vi "specu1a 1.0.0 Write User EEPROM.vi"(0 "Device Handle":i32, 1 "Address":u16, 2 "EEPROM String in":string, 3 "error in (no error)":errorcluster, 4 "Length":u16=256) -> (5 "Device Handle out":i32, 6 "EEPROM String out":string, 7 "error out":errorcluster)   [LabVIEW 2010]
uses:
  WINDOWS/SYSTEM32/DRIVERS/specu1a.dll
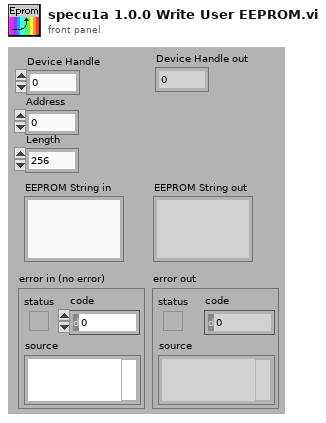
[diagram p1: front panel]
types:
  T1 = cluster{"[0]":u8, "[1]":u8, "[2]":u8, "[3]":u8, "[4]":u8, "[5]":u8, "[6]":u8, "[7]":u8, "[8]":u8, "[9]":u8, "[10]":u8, "[11]":u8, "[12]":u8, "[13]":u8, "[14]":u8, "[15]":u8, "[16]":u8, "[17]":u8, "[18]":u8, "[19]":u8, "[20]":u8, "[21]":u8, "[22]":u8, "[23]":u8, "[24]":u8, "[25]":u8, "[26]":u8, "[27]":u8, "[28]":u8, "[29]":u8, "[30]":u8, "[31]":u8, "[32]":u8, "[33]":u8, "[34]":u8, "[35]":u8, "[36]":u8, "[37]":u8, "[38]":u8, "[39]":u8, "[40]":u8, "[41]":u8, "[42]":u8, "[43]":u8, "[44]":u8, "[45]":u8, "[46]":u8, "[47]":u8, "[48]":u8, "[49]":u8, "[50]":u8, "[51]":u8, "[52]":u8, "[53]":u8, "[54]":u8, "[55]":u8, "[56]":u8, "[57]":u8, "[58]":u8, "[59]":u8, "[60]":u8, "[61]":u8, "[62]":u8, "[63]":u8}
  T2 = typedef "specu1a 1.0.0 Error codes.ctl" = enum16{"INVALID_HANDLE_VALUE", "USBDEV_SUCCESS", "USBDEV_INVALID_HANDLE", "USBDEV_UNSUCCESS", "USBDEV_INVALID_VALUE", "USBDEV_CHECK_NORMAL", "USBDEV_CHECK_INVALID", "USBDEV_CHECK_REMOVE", "USBDEV_CHECK_OTHER", "USBDEV_RESET_ERROR", "USBDEV_BULKSIZE_ERROR", "USBDEV_BULK_READ_ERROR", "USBDEV_BULK_NOT_UPDATED", "USBDEV_TIME_OVER_ERROR", "USBDEV_TIME_UNDER_ERROR", "USBDEV_TIME_SET_ERROR", "USBDEV_SET_GAIN_ERROR", "USBDEV_GET_TEMP_ERROR", "USBDEV_SET_TRIGGER_ERROR", "USBDEV_RW_EEP_ADDR_ERROR", "USBDEV_RW_EEP_SIZE_ERROR", "USBDEV_RW_EEP_OVER_ERROR", "USBDEV_RW_EEP_ERROR", "UNITID_PRODUCTID_CONFLICT", "UNKNOWN_ERROR"}
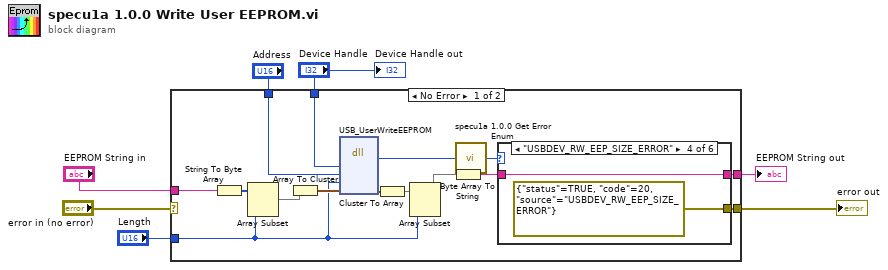
[diagram p0: block diagram]
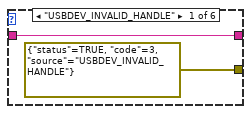
[diagram p2: hidden frame]
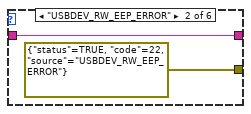
[diagram p3: hidden frame]
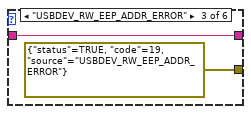
[diagram p4: hidden frame]
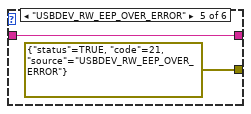
[diagram p5: hidden frame]
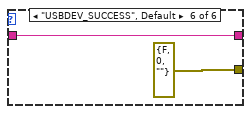
[diagram p6: hidden frame]
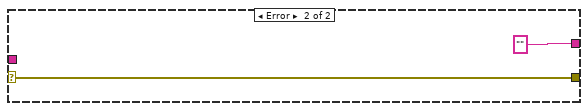
[diagram p7: hidden frame]
diagram:
  n1 = case shown="No Error" "error in (no error)" {
    selector: "error in (no error)" -> [_ w36]
    tunnel: [w21 w36] -> w6
    tunnel: "Device Handle" -> [w16 _]
    tunnel: "Address" -> [w15 _]
    tunnel: "Length" -> [w8 _]
    tunnel: [w17 "" ("string")] -> w1
    tunnel: "EEPROM String in" -> [w10 _]
    frame No Error {
      n2 = String To Byte Array(string=w10) -> (unsigned byte array=w11:u8[])
      n3 = Array Subset(array=w11, length=w8) -> (w9:u8[])  [unwired: 1 in]
      n4 = Array To Cluster(array=w9) -> (cluster=w14:T1)
      n5 = dll-call lib="C:/WINDOWS/SYSTEM32/DRIVERS/specu1a.dll" fn="USB_UserWriteEEPROM" label="1.0.0 Write User EEPROM"("Device Handle"=w16, "Address"=w15, "Length"=w8, w14) -> (w13:u16, w12:T1)  [unwired: 6 in, 2 out]
      n6 = Cluster To Array(cluster=w12) -> (array=w20:u8[])
      n7 = Array Subset(array=w20, length=w8) -> (w19:u8[])  [unwired: 1 in]
      n8 = Byte Array To String(unsigned byte array=w19) -> (string=w18:string)
      n9 = call "specu1a 1.0.0 Get Error Enum.vi"("Error Code in"=w13) -> ("Specu1a 1.0.0 Error code out"=w22:T2)  [unwired: 4 in]
      n10 = case shown="\"USBDEV_RW_EEP_SIZE_ERROR\"" w22 {
        tunnel: [w23 w25 w27 w29 w31 w33] -> w17
        tunnel: [errorcluster {"status"=TRUE, "code"=3, "source"="USBDEV_INVALID_HANDLE"} ("error out") errorcluster {"status"=TRUE, "code"=22, "source"="USBDEV_RW_EEP_ERROR"} ("error out") errorcluster {"status"=TRUE, "code"=19, "source"="USBDEV_RW_EEP_ADDR_ERROR"} ("error out") errorcluster {"status"=TRUE, "code"=20, "source"="USBDEV_RW_EEP_SIZE_ERROR"} ("error out") errorcluster {"status"=TRUE, "code"=21, "source"="USBDEV_RW_EEP_OVER_ERROR"} ("error out") errorcluster {"status"=FALSE, "code"=0, "source"=""} ("error out")] -> w21
        tunnel: w18 -> [w23 w25 w27 w29 w31 w33]
        frame "USBDEV_INVALID_HANDLE" {
        }
        frame "USBDEV_RW_EEP_ERROR" {
        }
        frame "USBDEV_RW_EEP_ADDR_ERROR" {
        }
        frame "USBDEV_RW_EEP_SIZE_ERROR" {
        }
        frame "USBDEV_RW_EEP_OVER_ERROR" {
        }
        frame "USBDEV_SUCCESS", Default {
        }
      }
    }
    frame Error {
    }
  }
  "error out" <- w6
  "EEPROM String out" <- w1
  "Device Handle out" <- "Device Handle"
